vi "Read Dashboard Variables.vi"() -> ()   [LabVIEW 2018]
uses:
  <vilib>/Rock Robotics/Network Tables/NT Read Number.vi
  Framework/Robot Global Data.vi
panel:
  out "Cheezy Drive Mode":u32=2
  out "Cargo Setpoint":dbl
  out "Elevator Duration":dbl
  out "Elevator Setpoint":dbl
  out "Pivot Right Setpoint":dbl
  out "Pivot Left Setpoint":dbl
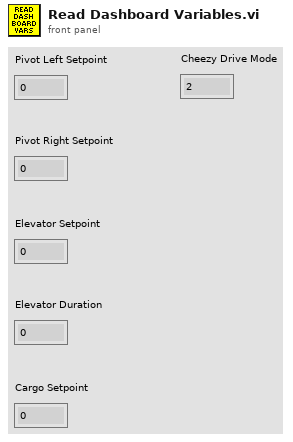
[diagram p1: front panel]
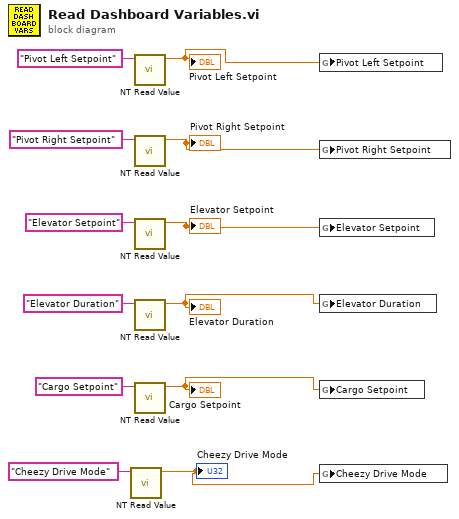
[diagram p0: block diagram]
diagram:
  n1 = call-poly <vilib>:"NT Read Value.vi"("Name"="Cheezy Drive Mode") -> ("Numeric"=w1:dbl)  [unwired: 9 in, 1 out]
  "Cheezy Drive Mode" <- w1
  n2 = call-poly <vilib>:"NT Read Value.vi"("Name"="Pivot Left Setpoint") -> ("Numeric"=w6:dbl)  [unwired: 9 in, 1 out]
  "Pivot Left Setpoint" <- w6
  n3 = call-poly <vilib>:"NT Read Value.vi"("Name"="Pivot Right Setpoint") -> ("Numeric"=w5:dbl)  [unwired: 9 in, 1 out]
  "Pivot Right Setpoint" <- w5
  n4 = call-poly <vilib>:"NT Read Value.vi"("Name"="Elevator Setpoint") -> ("Numeric"=w4:dbl)  [unwired: 9 in, 1 out]
  "Elevator Setpoint" <- w4
  n5 = call-poly <vilib>:"NT Read Value.vi"("Name"="Elevator Duration") -> ("Numeric"=w3:dbl)  [unwired: 9 in, 1 out]
  "Elevator Duration" <- w3
  n6 = call-poly <vilib>:"NT Read Value.vi"("Name"="Cargo Setpoint") -> ("Numeric"=w2:dbl)  [unwired: 9 in, 1 out]
  "Cargo Setpoint" <- w2
  n7 = global write "Robot Global Data.vi" "Pivot Left Setpoint"(w6) -> ()
  n8 = global write "Robot Global Data.vi" "Pivot Right Setpoint"(w5) -> ()
  n9 = global write "Robot Global Data.vi" "Elevator Setpoint"(w4) -> ()
  n10 = global write "Robot Global Data.vi" "Elevator Duration"(w3) -> ()
  n11 = global write "Robot Global Data.vi" "Cargo Setpoint"(w2) -> ()
  n12 = global write "Robot Global Data.vi" "Cheezy Drive Mode"(w1) -> ()
